vi "MintDAQ_Beta.vi"() -> ()   [LabVIEW 2016]
panel:
  in  "Cap 1":bool
  in  "Cap 2":bool
  in  "Freq":dbl=0.01
  in  "Amplitude 2":dbl
  in  "Amplitude":dbl=0.8
  in  "Freq":dbl=23.0
  in  "Write Rate":dbl=10.0 caption="dt"
  in  "Sampling Rate":dbl=40000.0
  in  "Buffer Size":i32=4000
  in  "Write":bool
  in  "?":T1(tab)=enum."Tiltmeters"
  out "Autocollimator":dynamicdata(graph)=[{"t0"=timestamp(3584301002.5607347 s since 1904-01-01), "dt"=0.001, "Y"=[0.43344412524716275, 0.44069982519207607, 0.43655847876988113, 0.42350642292314034, 0.4146197136070306, 0.40328027718902293, 0.39942297611809274, 0.4138427514859054, 0.43133329303091206, 0.4401128151072484, 0.43836303037775065, 0.4268035667025681, 0.41776134669103937, 0.4081520871618321, 0.3973264314407923, 0.40451695532239695, 0.42365021840797523, 0.4371180164475837, 0.44051733088947315, 0.43218711118964986, 0.4199243425497037, 0.41144729607965697, 0.40023572923979245, 0.40256453255522423, 0.4201710092812293, 0.43540959521302963, 0.44061842403674967, 0.43514094770763817, 0.4229076947032227, 0.41542396512922825, 0.4036505189077752, 0.39764993036831303, 0.41128629312723475, 0.42947942407640227, 0.4393467955648082, 0.439042631598667, 0.4271195679597182, 0.4169354468917369, 0.40734018701660385, 0.39899684628439686, 0.4082397862434385, 0.4262945383060813, 0.43778423869402877, 0.43953504788495423, 0.43013073777755223, 0.4190052781090954, 0.4114736084618774, 0.39912033284721876, 0.39913511226819326, 0.41637529988773103, 0.4326674073674492, 0.43974541690406393, 0.43570297775219, 0.4228391823041936, 0.4140567272130008, 0.402701353056287, 0.3991090457834896, 0.4137770345418973, 0.43097323181603453, 0.4394470896782597, 0.4377942918071419, 0.4263116695710484, 0.4171272850724305, 0.4075348167671378, 0.3970839223594497, 0.4044637556449303, 0.4233829165327582, 0.43680544817756956, 0.4402300393978032, 0.4319166495398041, 0.41960570181479623, 0.4111593303392392, 0.40019476380839447, 0.40300233950678993, 0.42065135304062434, 0.4355014297003315, 0.44083554591542506, 0.4351436898724957, 0.4227202848683051, 0.41516835962986626, 0.4036343684260499, 0.39781155478525676, 0.4113785124281454, 0.42957368340023233, 0.4395899330139984, 0.43921976442080857, 0.4276083237349742, 0.4171979089612628, 0.40734771090408123, 0.39878896340014114, 0.40840145058911986, 0.4268058170469636, 0.4388983111642708, 0.4406845835982937, 0.43145885626559677, 0.4203370587721238, 0.41243669736511696, 0.39995864936217074, 0.40047445740636817, 0.41809542489158874], "attributes"=variant("NI_ChannelName"=variant(string "Voltage_0 (Resampled)"), "NI_OriginalChannelName"=variant(string "Voltage_0"), "NI_UnitDescription"=variant(string "Volts"))}, {"t0"=timestamp(3584301002.5607347 s since 1904-01-01), "dt"=0.001, "Y"=[-0.4899930623675261, -0.49618517779377413, -0.49147473661274943, -0.47916473468257553, -0.4704209717410225, -0.4582103112231087, -0.4526439182566501, -0.4659935832899469, -0.48455155517052584, -0.49424384784604775, -0.4932876028975129, -0.4820006431763008, -0.4713454192343676, -0.46126420772334953, -0.4526272342865088, -0.4612194371103458, -0.4797607607514805, -0.49302166652545454, -0.49521427664385614, -0.4868851477690577, -0.47533904868769833, -0.46672055134251855, -0.4541546185640615, -0.45500585120320913, -0.47242507473390616, -0.48873125108294935, -0.4945101576910096, -0.4899985184460449, -0.47743833204721203, -0.4681475657146796, -0.4568603632196832, -0.45348452666153055, -0.4676122352684016, -0.4854852393103641, -0.49448520869432916, -0.4929760361070191, -0.48215125593273594, -0.4724288980813809, -0.46230160185882047, -0.45255984568019675, -0.4603440066276953, -0.4790831606691835, -0.49193190119468344, -0.4939058046810938, -0.485233635661633, -0.47322045802489393, -0.4644010543949078, -0.45350452925151147, -0.4555514886382289, -0.47263933075512876, -0.4889300758093243, -0.4950357596717817, -0.49031038481930594, -0.47827199879209714, -0.46999509979188464, -0.4577384596085571, -0.45219785195499623, -0.4659456404234807, -0.4845318190554642, -0.4940755974102945, -0.49312101619460347, -0.4816196861704534, -0.471090372935818, -0.46103550206715527, -0.45263650825676627, -0.46137101942036873, -0.4798528078286872, -0.49313741198078714, -0.49543043621354604, -0.48695040146175766, -0.4754215207234197, -0.4669228011335708, -0.45462597451738224, -0.455656611737308, -0.4731293161972794, -0.4894979885994622, -0.4952040342980257, -0.4902406511721809, -0.4774719474264416, -0.46846835181803426, -0.45710476738836775, -0.4538789376280827, -0.4679295376321548, -0.4857340010820316, -0.4952446398898893, -0.4941617238524955, -0.48283552180991424, -0.472828386804153, -0.46237264355045776, -0.45247223540877285, -0.4605043030686478, -0.4795100791768031, -0.4928472486855602, -0.4951132365031468, -0.4866591336331644, -0.4744833451831475, -0.4653165753980979, -0.45402960545544296, -0.4567301182540441, -0.47430536603009305], "attributes"=variant("NI_ChannelName"=variant(string "Voltage_1 (Resampled)"), "NI_OriginalChannelName"=variant(string "Voltage_1"), "NI_UnitDescription"=variant(string "Volts"))}, {"t0"=timestamp(3584301002.5607347 s since 1904-01-01), "dt"=0.001, "Y"=[0.4752534068648039, 0.4828089160742462, 0.4788214769070343, 0.46572582080473335, 0.4565461791038042, 0.4443905362197303, 0.44000211116761917, 0.45503506545430505, 0.4729492304645799, 0.48202113067256525, 0.4808637091287431, 0.46920339337455635, 0.459935061678949, 0.44976240866428896, 0.4380479127034327, 0.4452268064842056, 0.46481582898769525, 0.47880170342650535, 0.48264420637467514, 0.4743906358277276, 0.46191057491608306, 0.4530840898894057, 0.4412318111486498, 0.4435215400985711, 0.46159457744762983, 0.477019787853237, 0.48255506818894933, 0.4772042494056515, 0.4648366957946227, 0.4573035093760146, 0.4449690262346409, 0.4381851188092257, 0.4520426997895871, 0.4709815651668292, 0.48115794076123564, 0.48112845083648254, 0.4694327073406184, 0.45888006844449786, 0.4487109118407287, 0.4395954454135707, 0.4492612853971449, 0.46794570620513515, 0.4798195763650816, 0.48151531103537404, 0.4724718956854497, 0.46126640623768145, 0.4533215340906096, 0.4400094793568389, 0.43962361572182707, 0.45724133993585503, 0.47407933524264184, 0.4817390509485612, 0.47814826426104107, 0.46512671712574083, 0.4558880569960872, 0.4438023941344438, 0.43981420179845593, 0.45493875604870854, 0.47251009857461485, 0.48149700806397755, 0.4801525843124307, 0.46851761572489187, 0.4592185111821079, 0.449107151166732, 0.4377481013634747, 0.445126787340761, 0.4647276210890167, 0.4786996491590686, 0.4825017668160714, 0.47414042594077266, 0.4617773738849871, 0.4528292667611211, 0.44104227652050243, 0.44397723860813226, 0.46206847167797016, 0.47744680199800166, 0.482904801169116, 0.4773367538146408, 0.4648981271291952, 0.4572110463365532, 0.4447038387899914, 0.4381429239312602, 0.4521789849056913, 0.47116042336556857, 0.48153309131277666, 0.4816012687760707, 0.46984090928218913, 0.45923197895345846, 0.4488122671488527, 0.4395189501881836, 0.4492260144608356, 0.4683041316217303, 0.4807697375573159, 0.48295048700141024, 0.4739386073659291, 0.4626122471257542, 0.45423849004920125, 0.44080911543567924, 0.4410275575529489, 0.4590714921116883], "attributes"=variant("NI_ChannelName"=variant(string "Voltage_2 (Resampled)"), "NI_OriginalChannelName"=variant(string "Voltage_2"), "NI_UnitDescription"=variant(string "Volts"))}, {"t0"=timestamp(3584301002.5607347 s since 1904-01-01), "dt"=0.001, "Y"=[-0.46741716497017777, -0.47335196640769966, -0.4688101106381729, -0.45664050832791825, -0.448213130229613, -0.43623637113558433, -0.4302350320045326, -0.443538767561202, -0.4620528306577105, -0.47180156044258226, -0.4708179292756164, -0.45932138214803, -0.44882444701322133, -0.4389473643137334, -0.43021263768566703, -0.4389290270042119, -0.45719365582869087, -0.4703195255934425, -0.4725062586174858, -0.46412351904437593, -0.45266599902163945, -0.44452929290396437, -0.43224727493757303, -0.433114799318174, -0.45019875498394113, -0.46635052962592644, -0.4719961600068473, -0.46714017408877456, -0.4545566334501105, -0.4457455334827045, -0.4346493726108762, -0.43132205254719647, -0.44530002650432604, -0.46285119812847075, -0.47207996069808766, -0.47059195488018213, -0.45955848571273333, -0.4500080560551608, -0.4401595273597742, -0.4301296000567366, -0.43801005748286365, -0.4566340086643006, -0.46948052785402705, -0.4715299136445929, -0.46296642056819104, -0.4510050717407777, -0.4421868675692818, -0.4312254572681137, -0.43334469002882126, -0.4502249766779762, -0.4663893185758022, -0.4723950091453868, -0.4677093870036369, -0.4556402366748204, -0.44762001610851043, -0.43565467909521993, -0.43006135245785876, -0.4436904043107216, -0.4620902280747182, -0.47142412511475446, -0.47024445029591094, -0.4589520553752298, -0.4485546596952788, -0.43859895643507807, -0.4306030776532733, -0.4393468653762087, -0.45741650230252456, -0.4704208110651226, -0.47263895113144194, -0.46421030635564, -0.4527845970734405, -0.444608571264416, -0.432363860493319, -0.4334958061593289, -0.45081792059554604, -0.46707088362812127, -0.4726735792855328, -0.46757879668582364, -0.4548368413126195, -0.4460545704137894, -0.43474301847712926, -0.43137276244766654, -0.445408995733169, -0.46311295892705107, -0.4725715287342226, -0.47153021415590585, -0.4602416931812259, -0.45035976038962683, -0.44019822805303566, -0.4301401207313045, -0.438126286596999, -0.4570490190948041, -0.4702425601487558, -0.472657799778612, -0.4639172885988271, -0.45188581974347247, -0.44311506846835363, -0.43191775344563943, -0.43456605480841076, -0.45198857446235324], "attributes"=variant("NI_ChannelName"=variant(string "Voltage_3 (Resampled)"), "NI_OriginalChannelName"=variant(string "Voltage_3"), "NI_UnitDescription"=variant(string "Volts"))}]
  out "Interferometer":dynamicdata(graph)=[{"t0"=timestamp(3584301002.6527343 s since 1904-01-01), "dt"=0.001, "Y"=[0.006829190660454283, 0.006804074276043003, 0.006842802827010677, 0.0068415847383131246, 0.006839182378433872, 0.00685776770236201, 0.0068254281770467815, 0.00679490793515514, 0.006826136166008299, 0.006839250927218066, 0.006885744974215802, 0.006872920153230099, 0.0068459556593170635, 0.0067788572277271844, 0.006810908798271245, 0.006843586682920005, 0.006844003743632374, 0.006861160983203973, 0.006829789230096557, 0.006814916139960706, 0.006791236131882309, 0.006763083615057042, 0.006819530591850722, 0.006824557604947039, 0.006798398078015609, 0.006804774029728807, 0.0068032101016440956, 0.006765665610306133, 0.006752128475637698, 0.006839443300822217, 0.006760255089729292, 0.006741599354218663, 0.00678611945914091, 0.006790148597221571, 0.006765265780400054, 0.006733891478046875, 0.006749705918959564, 0.006678182149209056, 0.006674296646808111, 0.006718840100145775, 0.006716051786096207, 0.006700679563828491, 0.006744182507010799, 0.006789261097002876, 0.006718023450393194, 0.006733849047081241, 0.006768159078276218, 0.00670562987110903, 0.0067931254919439184, 0.006766590257329877, 0.006757634195636475, 0.006738605612389788, 0.006738138892240513, 0.0067589991043940836, 0.006799606400498515, 0.006810258091940859, 0.006745698101846311, 0.0067758918641107795, 0.0067580007161438735, 0.006784504446825061, 0.0067947629744846885, 0.006759420468503427, 0.006807751744288853, 0.006844330204419778, 0.006796933133234253, 0.006767604642546505, 0.006800642686309006, 0.00680934660333741, 0.006797574852825216, 0.006818358205769789, 0.006796135078595576, 0.006797976710975998, 0.00682167125723123, 0.0068453855491922636, 0.00683078505894028, 0.006816237213630237, 0.006836766164359942, 0.006830055877761378, 0.006809951504255314, 0.006879278069927046, 0.006828506557633108, 0.006796904922860819, 0.00678984148192317, 0.0068003542314009615, 0.006781409933802676, 0.006768389062226075, 0.0068260796398966535, 0.006782028912536799, 0.006763515121172703, 0.006736620043527606, 0.0067113376652639615, 0.006758038372946205, 0.006762727514682312, 0.006764384225255027, 0.006715498251011387, 0.006724243652234973, 0.0066958975856384, 0.006695695525440389, 0.0067368957309638785, 0.006717783312505214], "attributes"=variant("NI_ChannelName"=variant(string "Voltage_0 (Resampled)"), "NI_OriginalChannelName"=variant(string "Voltage_0"), "NI_UnitDescription"=variant(string "Volts"))}, {"t0"=timestamp(3584301002.6527343 s since 1904-01-01), "dt"=0.001, "Y"=[0.014079520299369902, 0.014089443536113735, 0.01413838279236252, 0.014073268951156152, 0.01406504585971624, 0.014094152205166504, 0.014076717713778275, 0.01410976032104998, 0.014083340578053195, 0.014083047059254608, 0.014073947149022274, 0.014145253440018832, 0.014094260993791834, 0.0140712503491944, 0.014059874273873623, 0.01405289434036577, 0.014047340666948032, 0.01409862304928333, 0.0140780703598332, 0.014092916485748829, 0.01404770682724726, 0.014088107561823415, 0.014062112790610122, 0.014041402834955993, 0.014071921491964982, 0.014043025726374177, 0.014073195489615439, 0.014063407668480674, 0.014092498018178494, 0.014058393522085606, 0.01405821946350781, 0.014034068491767523, 0.014046707469062806, 0.014052762554210126, 0.014121276368777845, 0.01407928275169214, 0.014016736267355124, 0.014002637471172086, 0.014004770641207642, 0.014010865997918256, 0.014038106702091477, 0.014000388730206906, 0.014003110570523036, 0.014035772574007713, 0.014015678283132122, 0.013995996432146158, 0.014014366493847085, 0.01402938421206668, 0.014017085207530632, 0.014054635185166007, 0.014038340870197532, 0.014069513721362708, 0.014031123864759243, 0.01402892779888155, 0.014061224413235873, 0.01404060636115332, 0.014044978845244149, 0.013997494228631023, 0.014071469993759932, 0.014062308683913503, 0.014075231637268865, 0.014074931537452704, 0.014091680839285385, 0.014096028326234987, 0.01412212044842212, 0.014084767395675726, 0.014031174341889817, 0.014017825746510044, 0.014019425281673164, 0.014027138319086589, 0.01401270152711483, 0.014097329823873036, 0.014108779023646675, 0.014042530650638322, 0.014032682296044144, 0.014098057535918914, 0.014032398902387104, 0.014054667811692102, 0.014052980427935688, 0.01412931155397704, 0.014098718955442072, 0.014095034956812436, 0.014049628590867239, 0.014093437040998746, 0.014071326434821394, 0.014055944856256063, 0.01402078171243926, 0.014052632057341656, 0.014048405726922885, 0.014081409428061308, 0.014003006477915724, 0.014049046467740472, 0.014007229224388525, 0.014063501022372934, 0.014139246375744385, 0.014061430667785901, 0.014079495475464476, 0.014006584025108057, 0.014038461617348556, 0.014020381795830343], "attributes"=variant("NI_ChannelName"=variant(string "Voltage_1 (Resampled)"), "NI_OriginalChannelName"=variant(string "Voltage_1"), "NI_UnitDescription"=variant(string "Volts"))}]
  out "Y-Tilt":dynamicdata(graph)
  out "X-Tilt":dynamicdata(graph)
  out "Interferometer Angle":dynamicdata(graph)=[{"t0"=timestamp(3584301002.652747 s since 1904-01-01), "dt"=0.001, "Y"=[0.014079523842758108, 0.01408882108377099, 0.014139037672450625, 0.01407280813247636, 0.014064729768797652, 0.014093702444871162, 0.014076359649149703, 0.01411085646219041, 0.014083787524917802, 0.014082287987847044, 0.014074911580000458, 0.014144148120125894, 0.01409290939216138, 0.014071860270478593, 0.014057498877325273, 0.014053501645067348, 0.014047463627659731, 0.014099356512726424, 0.0140787455400635, 0.01409152835182853, 0.014049362307693625, 0.014087897830537143, 0.0140614757950326, 0.014042240804392111, 0.014070969369652558, 0.014044862257688149, 0.014073507734953052, 0.014063096601953953, 0.014092704610592833, 0.014057846494315143, 0.014057636810089123, 0.014033601584274325, 0.014047269712564809, 0.014054091284079504, 0.014121881593934958, 0.014078136875977384, 0.014017481543910942, 0.014002358090528645, 0.01400554546932183, 0.014010414955054694, 0.014038264896493648, 0.013999825279258285, 0.01400260275898491, 0.01403404230826596, 0.014015566872301042, 0.01399606172889438, 0.01401524513663883, 0.01402868894874523, 0.014017869341953869, 0.014053872816437472, 0.014039558372932455, 0.014068713483619042, 0.014032643875552408, 0.01402809579860335, 0.014061676497261831, 0.014041263242768722, 0.014044765126358884, 0.013998027952526065, 0.014072116056769167, 0.014062055203707482, 0.014076231461729122, 0.014075052887551096, 0.014091733649736803, 0.014096658086670839, 0.014121966803459183, 0.014085631910137323, 0.014030455531931753, 0.014017122443594274, 0.01401924157308815, 0.014027275362907635, 0.014013742246393297, 0.014098782021426151, 0.014108111501473146, 0.01404194075891019, 0.014033749910072535, 0.01409771047400392, 0.014031347764116115, 0.014054660423562678, 0.014053518858002158, 0.014129918899766608, 0.01409814111093245, 0.014094692849691937, 0.014049505711538837, 0.014094509569479151, 0.014072003851555298, 0.01405603645142166, 0.014020787548272127, 0.014051507739459205, 0.01404965592418739, 0.014080831673375952, 0.01400344836335159, 0.014048947686481078, 0.014007080419140387, 0.014064113346367164, 0.014138793541416384, 0.014060465784733089, 0.014079431005924018, 0.01400604029938445, 0.014038771619406138, 0.01402036849841128], "attributes"=variant("NI_ChannelName"=variant(string "Voltage_1 (Resampled)"), "NI_OriginalChannelName"=variant(string "Voltage_1"), "NI_UnitDescription"=variant(string "Volts"))}]
  out "Autocollimator Angle":dynamicdata(graph)=[{"t0"=timestamp(3584301002.5607347 s since 1904-01-01), "dt"=0.001, "Y"=[-0.05451833877723473, -0.05477533979676578, -0.05480582827131981, -0.054733234251106065, -0.05438452166115732, -0.05328249062231282, -0.05282928135642799, -0.05380742715640242, -0.05429267469512887, -0.05453029541879096, -0.055158108535643346, -0.05495324117150584, -0.054737105032500843, -0.05390617367682065, -0.05287580869831008, -0.053150091215801595, -0.05375844613293926, -0.054305489087989864, -0.05474256186511284, -0.05468787010309875, -0.054464146880406406, -0.053980763474418665, -0.05319596601622297, -0.05341507708546636, -0.05409286356894648, -0.05423308435586057, -0.05452651489614367, -0.05453725909672287, -0.05437428211257543, -0.05433893468520682, -0.053531422557000344, -0.052740294552652806, -0.053250414130049384, -0.05415371986656394, -0.05442042116671404, -0.05463111639248197, -0.05482945152523553, -0.05442711090661558, -0.053612604169809015, -0.05276062517907868, -0.05356674134825469, -0.054364647974460806, -0.05473078730661945, -0.054529266336172895, -0.054872106202178986, -0.05484029684965096, -0.05424943872507388, -0.053020503666677266, -0.05278046062927735, -0.05338179240033376, -0.05399934610464124, -0.05462878331890356, -0.0550440444000253, -0.05482138827862627, -0.0542636140340086, -0.053271217757039795, -0.05299800290380298, -0.0537637882823139, -0.054184528206733, -0.05471748678812945, -0.05496820360224187, -0.05470350277314279, -0.05463311899197042, -0.05386273864045209, -0.052807622422947814, -0.053089720433317195, -0.0539894738939846, -0.05458084492323193, -0.05492879411526293, -0.05471494807201495, -0.05470264547182372, -0.05401921708034396, -0.053004545381501254, -0.05344398804351714, -0.05408676006037784, -0.054669368635636456, -0.05469729224640852, -0.05470551107247462, -0.05470159312764469, -0.054550536191225144, -0.053211554910672726, -0.05248128758956602, -0.05330129496244606, -0.054265667488309556, -0.054598057744387876, -0.05501212395163068, -0.054721672453989546, -0.05453950323691921, -0.053729192585936156, -0.05293366875685083, -0.05331091185378958, -0.05417210090301452, -0.05452392463979469, -0.05490399470516479, -0.05505330134879471, -0.05485221959895576, -0.05418344956409292, -0.05297257260307909, -0.052866907118601585, -0.053531331100620604], "attributes"=variant("NI_ChannelName"=variant(string "Voltage_0 (Resampled)"), "NI_OriginalChannelName"=variant(string "Voltage_0"), "NI_UnitDescription"=variant(string "Volts"))}, {"t0"=timestamp(3584301002.5607347 s since 1904-01-01), "dt"=0.001, "Y"=[0.029184874400107766, 0.029669964725631895, 0.02960380431772896, 0.029435387639123962, 0.028980595921586996, 0.028729684540872866, 0.02907643674907737, 0.028940253349997197, 0.029047499543346057, 0.029121962095730525, 0.02928959942345358, 0.029655428059348773, 0.02938076977263026, 0.029178858486904546, 0.02915843360419281, 0.02875499375154043, 0.029106053892906436, 0.029415157932796126, 0.029558825682914916, 0.029748360244639466, 0.02959070887957728, 0.02900148552377682, 0.02859649573632491, 0.028310538126707523, 0.028644755566355724, 0.028940618187186348, 0.029250973456318403, 0.02985522336081171, 0.02990198150552743, 0.029240394970527935, 0.02901526563556768, 0.02873266721257002, 0.028754890186645187, 0.0292319062945649, 0.029087666241611947, 0.029182614070472436, 0.029528950578401207, 0.029237856496264477, 0.028956988429858374, 0.02920088778390613, 0.02882022760087491, 0.028949607052927588, 0.029094541405657818, 0.02912515043959512, 0.029120149635372572, 0.02900584976595074, 0.029022158842350463, 0.029053830542728892, 0.028718292497503038, 0.028892094164828703, 0.029149335140592206, 0.029417217514454235, 0.029514935252490913, 0.029565372123483882, 0.02919480164175955, 0.02887630452485412, 0.028722341227765128, 0.028675323472041703, 0.02897489544084521, 0.029392663289044496, 0.029824842326365376, 0.029637602227388652, 0.029397921351316653, 0.029331664893484953, 0.028662183913639065, 0.028415707636525275, 0.02893622093302352, 0.029429922855068385, 0.029665115737803532, 0.02972935630931994, 0.029547017836511737, 0.029165487232220108, 0.029055439836962058, 0.028655078231310156, 0.0287494884170076, 0.029010425976667573, 0.02928174068810139, 0.02959849853901873, 0.029571964958395675, 0.02925007905005125, 0.02921046706117887, 0.029185359628159907, 0.029032417421852738, 0.02921238635610886, 0.029425074046687212, 0.02950823327882449, 0.029541908662657133, 0.02930095588686082, 0.02900602253337073, 0.029065631981068485, 0.028872004576206735, 0.028962479142700916, 0.02928555170258849, 0.029224339721921764, 0.029737732695260113, 0.029505716148848084, 0.02901709012437195, 0.02883814858127603, 0.028648014906134667, 0.028758078332581812], "attributes"=variant("NI_ChannelName"=variant(string "Voltage_3 (Resampled)"), "NI_OriginalChannelName"=variant(string "Voltage_3"), "NI_UnitDescription"=variant(string "Volts"))}]
  in  "PID Input":bool
  out "Feedback":dynamicdata(graph)=[{"t0"=timestamp(3584301002.560747 s since 1904-01-01), "dt"=0.001, "Y"=[0.0, 0.0, 0.0, 0.0, 0.0, 0.0, 0.0, 0.0, 0.0, 0.0, 0.0, 0.0, 0.0, 0.0, 0.0, 0.0, 0.0, 0.0, 0.0, 0.0, 0.0, 0.0, 0.0, 0.0, 0.0, 0.0, 0.0, 0.0, 0.0, 0.0, 0.0, 0.0, 0.0, 0.0, 0.0, 0.0, 0.0, 0.0, 0.0, 0.0, 0.0, 0.0, 0.0, 0.0, 0.0, 0.0, 0.0, 0.0, 0.0, 0.0, 0.0, 0.0, 0.0, 0.0, 0.0, 0.0, 0.0, 0.0, 0.0, 0.0, 0.0, 0.0, 0.0, 0.0, 0.0, 0.0, 0.0, 0.0, 0.0, 0.0, 0.0, 0.0, 0.0, 0.0, 0.0, 0.0, 0.0, 0.0, 0.0, 0.0, 0.0, 0.0, 0.0, 0.0, 0.0, 0.0, 0.0, 0.0, 0.0, 0.0, 0.0, 0.0, 0.0, 0.0, 0.0, 0.0, 0.0, 0.0, 0.0, 0.0], "attributes"=variant("NI_ChannelName"=variant(string "Voltage_0 (Resampled)"), "NI_OriginalChannelName"=variant(string "Voltage_0"), "NI_UnitDescription"=variant(string "Volts"))}, {"t0"=timestamp(3584301002.560747 s since 1904-01-01), "dt"=0.001, "Y"=[-0.003049692667419053, -0.0030011632054061078, -0.002996518018028922, -0.0029827779629064987, -0.002969936113352624, -0.0029686840885194002, -0.0030714550816880013, -0.0031182601097152316, -0.0030961181067506215, -0.0030702960683242127, -0.0031556696339665167, -0.003056010712971206, -0.0029590470292609763, -0.0030446429366765533, -0.002998755886991544, -0.00289757201639633, -0.0029364950409000007, -0.0029978703214920866, -0.0030534579761776716, -0.00306865013859312, -0.003013746188494248, -0.002941985739241768, -0.002975215182450896, -0.0030736031997608475, -0.0031436370132216385, -0.003119638151751415, -0.00313688360069503, -0.003200363446943197, -0.003120515838852851, -0.0030992073779693096, -0.0030333548858917413, -0.002935256533575503, -0.002944937708864363, -0.003008774658902448, -0.0030689687797508373, -0.0030487168992998507, -0.003080560232342409, -0.002976009922175736, -0.002990476808699664, -0.002997972161262606, -0.0031482346201067296, -0.003215133385025752, -0.0031569483922634775, -0.003123058031455838, -0.0030834162651266045, -0.0031345660821078913, -0.0031593501896138776, -0.0030466035459227356, -0.0029823811664562356, -0.002966955667432815, -0.0030550137544457373, -0.0030121888939130233, -0.0030919653304827713, -0.0030764282655193578, -0.0030286548502291193, -0.002962715438738431, -0.0030469850748333807, -0.003143821683320151, -0.0031858434346675522, -0.0032726993185585433, -0.0031859175661686366, -0.0030983549242839655, -0.003126499096708473, -0.003154439027166124, -0.003051078595666944, -0.0029192029414693726, -0.0029795320910118933, -0.0030517968700238566, -0.0031078090437984766, -0.0030798043887342646, -0.002968772323109508, -0.00299256205978614, -0.0029752696012527694, -0.003065746078914158, -0.003142664871777985, -0.0031278285009034177, -0.003102616171912688, -0.003078624786513096, -0.003012176456560062, -0.0030685407894212925, -0.0030532677393301797, -0.0029440112864748194, -0.002839468055274482, -0.002955781919963107, -0.0030284792855605597, -0.002991621109287228, -0.0029662293652921628, -0.002934837279029464, -0.0029292499538955707, -0.0030142614762774973, -0.003142299723375851, -0.003094740857359699, -0.0030834498434977623, -0.003223813466166711, -0.0031622302883786233, -0.0031387689775952765, -0.0031624680902710553, -0.0030453733210472913, -0.002927372808287793, -0.00292036287756316], "attributes"=variant("NI_ChannelName"=variant(string "Voltage_4 (Resampled)"), "NI_OriginalChannelName"=variant(string "Voltage_4"), "NI_UnitDescription"=variant(string "Volts"))}, {"t0"=timestamp(3584301002.560747 s since 1904-01-01), "dt"=0.001, "Y"=[-0.0419451691736932, -0.04213397136367565, -0.042154391527895005, -0.04210039078733851, -0.04182406066280207, -0.040979425792335815, -0.04064575377650065, -0.04139845227224993, -0.04176552138001907, -0.041945875961085045, -0.04243495974688696, -0.04226950687152701, -0.04210445195558116, -0.04145475774024459, -0.04066738340557622, -0.04089095505973653, -0.041358847359998896, -0.041777527551470586, -0.042112761651914514, -0.04206654782148995, -0.041894063161484134, -0.04151425860188682, -0.04091468488219391, -0.041094128540214436, -0.0416144467008395, -0.04172172418310117, -0.041947643195890415, -0.04194504450699992, -0.04182399360111914, -0.04179189205963497, -0.041163298556466596, -0.04057226839332534, -0.040978484135791055, -0.04165521719640903, -0.041858489248501815, -0.042031969991565735, -0.04218032531260918, -0.04186697616857548, -0.041234925560187874, -0.0405799882220148, -0.041213879051893006, -0.04182506713537269, -0.042103762388083624, -0.04194632157334728, -0.042210231513215186, -0.04218009548111838, -0.04171713802069411, -0.040776902708704585, -0.04060867978652026, -0.041068744876227914, -0.04154361184666005, -0.04202848435433248, -0.042339163200905285, -0.04216588353396274, -0.04172787504367163, -0.040970386899929136, -0.040773365430044256, -0.04136304511733595, -0.041680931600763915, -0.04209776762485897, -0.04228342224083276, -0.04208181131018098, -0.04202843973054086, -0.0414254571804388, -0.04061494371421473, -0.04084394783327905, -0.041536638588880716, -0.04199400353439718, -0.042252954133303974, -0.04207980125627409, -0.04207292445054595, -0.041536161358252374, -0.04076991367817173, -0.04111832681371705, -0.04161322424789044, -0.04205551755409712, -0.04207491976463538, -0.04208079558385167, -0.042083216024666845, -0.04195632537604731, -0.04091868940555001, -0.04037317065188369, -0.041012020891848855, -0.041748708262008515, -0.04199883176583878, -0.04231918945121469, -0.042091065524704735, -0.04195788335179344, -0.04132179219068758, -0.04071692878925155, -0.04101304361525849, -0.04167341611429567, -0.04194659385006853, -0.042237546018531275, -0.04234773554837193, -0.042185084170227025, -0.04166361582372886, -0.04073714289884529, -0.040668900705412944, -0.0411887905747883], "attributes"=variant("NI_ChannelName"=variant(string "Voltage_0 (Resampled)"), "NI_OriginalChannelName"=variant(string "Voltage_0"), "NI_UnitDescription"=variant(string "Volts"))}, {"t0"=timestamp(3584301002.552747 s since 1904-01-01), "dt"=0.001, "Y"=[4.698558856944605e-06, 4.7042384185892055e-06, 4.675162549090393e-06, 4.689973323617886e-06, 4.6985804343707245e-06, 4.676409797307714e-06, 4.674852774949815e-06, 4.688802233997341e-06, 4.6912806572878e-06, 4.690052524075735e-06, 4.681342348104294e-06, 4.678288592925336e-06, 4.681037573939893e-06, 4.677931232195188e-06, 4.667534564698385e-06, 4.680664590919649e-06, 4.6924544748470255e-06, 4.670149948052578e-06, 4.670062309599805e-06, 4.676237222652673e-06, 4.666492909656395e-06, 4.6804157105122615e-06, 4.6871886831658706e-06, 4.6787444183540155e-06, 4.672749559758632e-06, 4.683738872036577e-06, 4.6630077375608405e-06, 4.657977036848412e-06, 4.676340571461413e-06, 4.700874197495369e-06, 4.69200456093008e-06, 4.698196222124365e-06, 4.685753924719665e-06, 4.682616863715975e-06, 4.678037258424881e-06, 4.6856936824801385e-06, 4.7020659695103085e-06, 4.682897907354301e-06, 4.702471991743499e-06, 4.685270732225905e-06, 4.6917773107079e-06, 4.6916108775713556e-06, 4.693880730462773e-06, 4.690245176248893e-06, 4.672587950542629e-06, 4.697889535228499e-06, 4.683440396462663e-06, 4.682546730759722e-06, 4.6916164315831145e-06, 4.683864725528507e-06, 4.697409380132391e-06, 4.6925340752527e-06, 4.691584514214445e-06, 4.6836452723541905e-06, 4.695694088268158e-06, 4.709697290250545e-06, 4.722568503764702e-06, 4.7009524756229445e-06, 4.685173101074728e-06, 4.682051079532445e-06, 4.701712532936734e-06, 4.682410760440411e-06, 4.683050718689626e-06, 4.663164494552434e-06, 4.687304587659254e-06, 4.695406112983935e-06, 4.680414416178407e-06, 4.69271982243097e-06, 4.689941558326997e-06, 4.689449896781862e-06, 4.69285229094534e-06, 4.679673743466315e-06, 4.6476534139927996e-06, 4.689067834928844e-06, 4.681949206553395e-06, 4.685045298025742e-06, 4.6860997041393756e-06, 4.666862811141036e-06, 4.655141263915157e-06, 4.667922440507146e-06, 4.663433957466344e-06, 4.677111243641375e-06, 4.6824597756597946e-06, 4.674640984086689e-06, 4.678432130249666e-06, 4.676092881061438e-06, 4.676925942360813e-06, 4.678860099784647e-06, 4.699454912900034e-06, 4.685755486753241e-06, 4.6874190169299055e-06, 4.680411876400209e-06, 4.69027949451859e-06, 4.68449302010556e-06, 4.677802336615631e-06, 4.707526014456434e-06, 4.689532594658673e-06, 4.691874093945714e-06, 4.678165342537276e-06, 4.70558607300561e-06], "attributes"=variant("NI_ChannelName"=variant(string "Voltage_1 (Resampled)"), "NI_OriginalChannelName"=variant(string "Voltage_1"), "NI_UnitDescription"=variant(string "Volts"))}]
  in  "Offset 1":dbl
  in  "Offset 2":dbl
  in  "AC Setpoint":dbl=-0.014
  in  "Gain":dbl
  in  "I term":dbl=0.01
  in  "Reset Button":bool
  in  "D term":dbl=60.0
  in  "Int Setpoint":dbl=0.00135
  # "Swing\nInjection"
  # "Torsion\nInjection"
  # "Interferometer"
  # "Autocollimator"
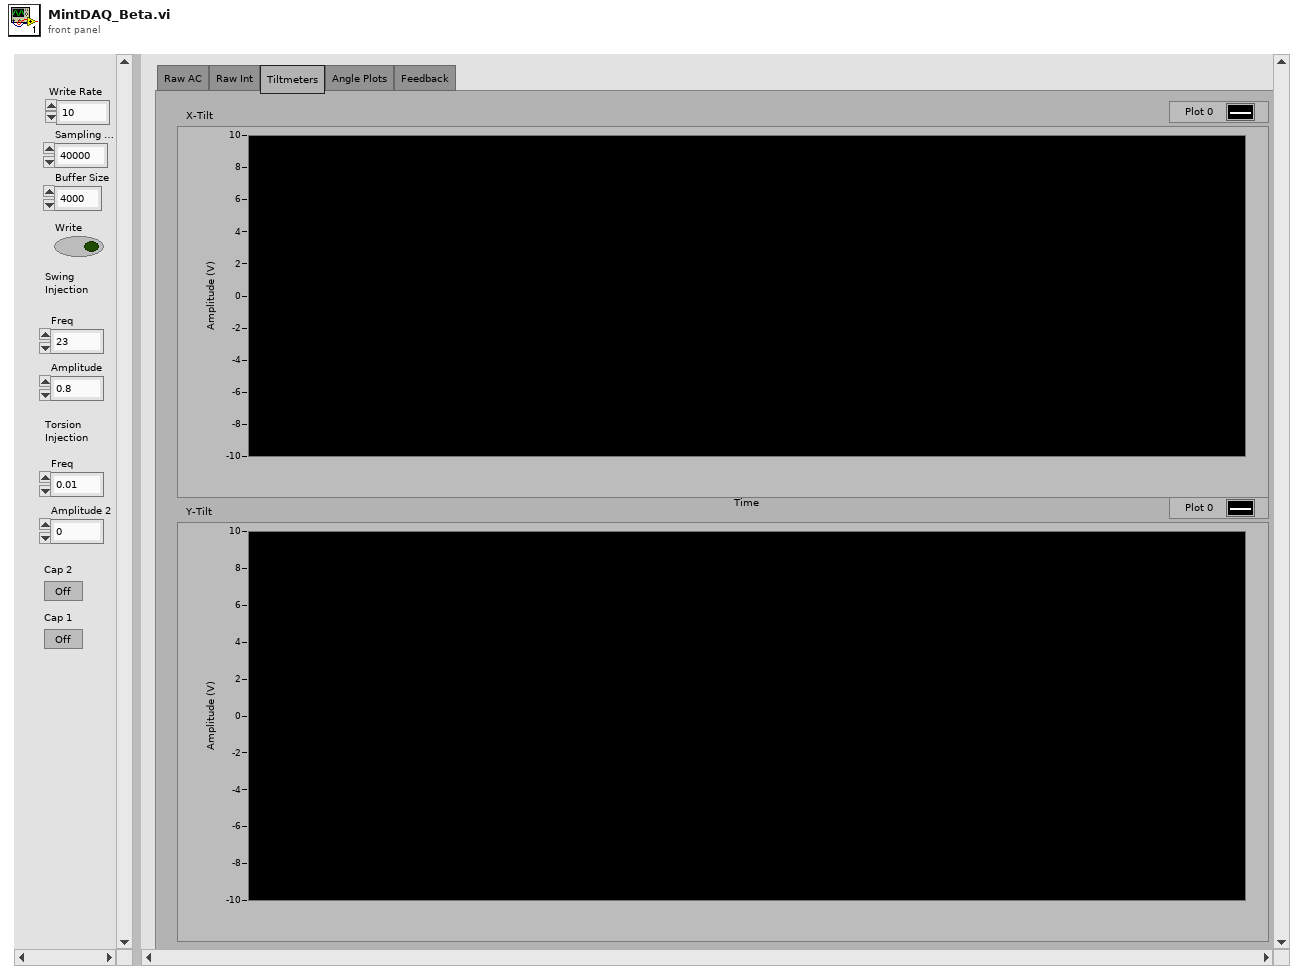
[diagram p1: front panel]
types:
  T1 = enum32{"Raw AC", "Raw Int", "Tiltmeters", "Angle Plots", "Feedback"}
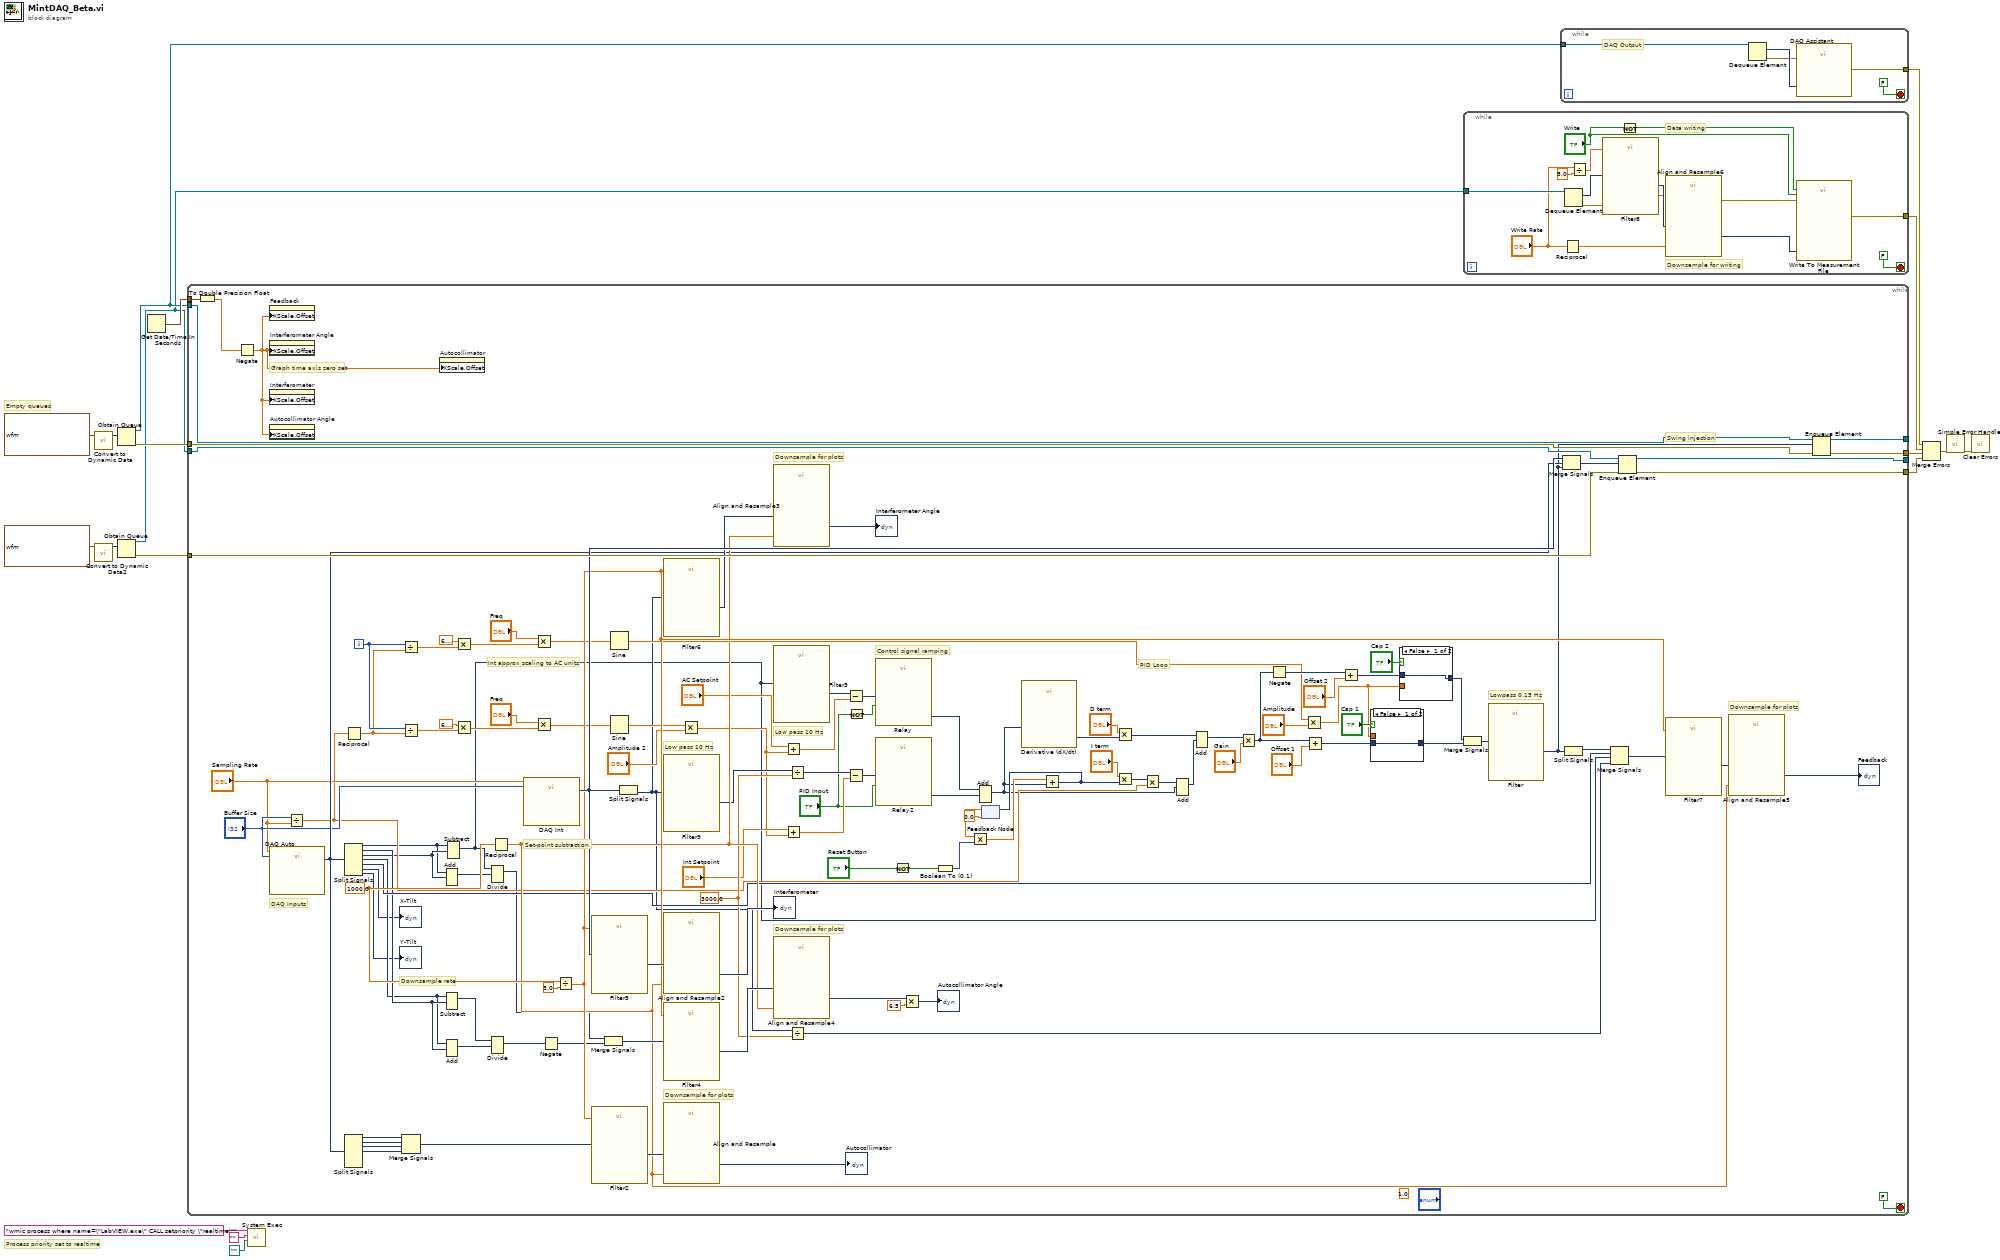
[diagram p0: block diagram]
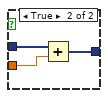
[diagram p2: hidden frame]
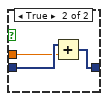
[diagram p3: hidden frame]
diagram:
  # "Empty queues"
  # "Process priority set to realtime"
  n1 = call "Convert to Dynamic Data"("Waveform"=waveform(dbl) {"t0"=timestamp(0 s since 1904-01-01), "dt"=1.0, "Y"=[]}) -> ("Dynamic Data Type"=w16:dynamicdata)  [unwired: 3 in]
  n2 = call "Convert to Dynamic Data2"("Waveform"=waveform(dbl) {"t0"=timestamp(0 s since 1904-01-01), "dt"=1.0, "Y"=[]}) -> ("Dynamic Data Type"=w14:dynamicdata)  [unwired: 3 in]
  n3 = Obtain Queue(element data type=w16) -> (queue out=w11:refnum<queue>, error out=w13:errorcluster)  [unwired: 4 in, 1 out]
  n4 = Obtain Queue(element data type=w14) -> (queue out=w10:refnum<queue>, error out=w12:errorcluster)  [unwired: 4 in, 1 out]
  n5 = Get Date/Time In Seconds() -> (seconds since 1Jan1904=w18:timestamp)
  n6 = while {
    tunnel: w18 -> [w136]
    tunnel: w11 -> [w133]
    tunnel: [w132] -> _
    tunnel: w10 -> [w116]
    tunnel: [w115] -> _
    tunnel: w13 -> [w114]
    tunnel: w12 -> [w113]
    tunnel: [w112] -> w8
    tunnel: [w111] -> w9
    i -> [w56]
    stop <- FALSE stop-if-true
    (unwired) 1.0 ("y")
    w92 = 3000.0 ("y")
    w96 = 1000.0 ("dt")
    # "Downsample for plots"
    # "Lowpass 0.15 Hz"
    # "PID Loop"
    # "Control signal ramping"
    # "Swing injection"
    # "Downsample rate"
    # "Downsample for plots"
    # "Downsample for plots"
    # "Downsample for plots"
    # "Int approx scaling to AC units"
    # "Set-point subtraction"
    # "Low pass 10 Hz"
    # "Low pass 10 Hz"
    # "DAQ Inputs"
    # "Graph time axis zero set"
    n7 = To Double Precision Float(number=w136) -> (double precision float=w135:dbl)
    n8 = Negate(x=w135) -> (-x=w134:dbl)
    n9 = property on="Feedback" class="WFChart (strict)"("XScale.Offset"=w134) -> ()  [unwired: 2 in, 2 out]
    n10 = property on="Interferometer Angle" class="WFChart (strict)"("XScale.Offset"=w134) -> ()  [unwired: 2 in, 2 out]
    n11 = property on="Interferometer" class="WFChart (strict)"("XScale.Offset"=w134) -> ()  [unwired: 2 in, 2 out]
    n12 = property on="Autocollimator Angle" class="WFChart (strict)"("XScale.Offset"=w134) -> ()  [unwired: 2 in, 2 out]
    n13 = call "DAQ Auto"("rate"="Sampling Rate", "number of samples"="Buffer Size") -> ("data"=w78:dynamicdata)  [unwired: 14 in, 3 out]
    n14 = Divide(x="Buffer Size", y="Sampling Rate") -> (x/y=w61:dbl)
    n15 = Split Signals(w78) -> (w83:dynamicdata, w82:dynamicdata, w81:dynamicdata, w80:dynamicdata)  [unwired: 7 in, 3 out]
    n16 = Split Signals(w78) -> (w26:dynamicdata, w31:dynamicdata, w27:dynamicdata, w30:dynamicdata, w94:dynamicdata, →"X-Tilt":dynamicdata, →"Y-Tilt":dynamicdata)  [unwired: 7 in]
    n17 = Reciprocal(x=w61) -> (1/x=w55:dbl)
    n18 = Divide(x=w56, y=w55) -> (x/y=w71:dbl)
    n19 = Divide(x=w56, y=w55) -> (x/y=w57:dbl)
    n20 = Merge Signals(w83, w82, w81, w80) -> (w79:dynamicdata)
    n21 = property on="Autocollimator" class="WFChart (strict)"("XScale.Offset"=w134) -> ()  [unwired: 2 in, 2 out]
    n22 = Add(1:w27, 2:w26) -> (0:w25:dynamicdata)  [unwired: 1 in, 1 out]
    n23 = Subtract(1:w31, 2:w30) -> (0:w28:dynamicdata)  [unwired: 1 in, 1 out]
    n24 = Add(1:w31, 2:w30) -> (0:w29:dynamicdata)  [unwired: 1 in, 1 out]
    n25 = Subtract(1:w27, 2:w26) -> (0:w21:dynamicdata)  [unwired: 1 in, 1 out]
    n26 = Multiply(x=6.283185307179586, y=w71) -> (x*y=w70:dbl)
    n27 = Multiply(x=6.283185307179586, y=w57) -> (x*y=w58:dbl)
    n28 = Divide(1:w25, 2:w21) -> (0:w24:dynamicdata)  [unwired: 1 in, 1 out]
    n29 = Divide(1:w29, 2:w28) -> (0:w23:dynamicdata)  [unwired: 1 in, 1 out]
    n30 = Reciprocal(x=w96) -> (1/x=w95:dbl)
    n31 = call "DAQ Int"("rate"="Sampling Rate", "number of samples"="Buffer Size") -> ("data"=w102:dynamicdata)  [unwired: 14 in, 3 out]
    n32 = Multiply(x="Freq", y=w70) -> (x*y=w68:dbl)
    n33 = Multiply(x="Freq", y=w58) -> (x*y=w59:dbl)
    n34 = Negate(x=w23) -> (-x=w22:dynamicdata)
    n35 = Divide(x=w96, y=3.0) -> (x/y=w97:dbl)
    n36 = call "Filter5"("Lower Cut-Off"=w97, "Signal"=w102) -> ("Filtered Signal"=w101:dynamicdata)  [unwired: 8 in, 1 out]
    n37 = call "Filter2"("Lower Cut-Off"=w97, "Signal"=w79) -> ("Filtered Signal"=w105:dynamicdata)  [unwired: 8 in, 1 out]
    n38 = Merge Signals(w24, w22) -> (w104:dynamicdata)
    n39 = Sine(x=w68) -> (sin(x)=w67:dbl)
    n40 = Sine(x=w59) -> (sin(x)=w60:dbl)
    n41 = Split Signals(w102) -> (w51:dynamicdata)  [unwired: 2 in, 1 out]
    n42 = call "Filter6"("Lower Cut-Off"=w97, "Signal"=w51) -> ("Filtered Signal"=w100:dynamicdata)  [unwired: 8 in, 1 out]
    n43 = call "Filter9"("Signal"=w51) -> ("Filtered Signal"=w50:dynamicdata)  [unwired: 9 in, 1 out]
    n44 = call "Align and Resample2"("dt"=w95, "Signals"=w101) -> ("Resampled Signals"=→"Interferometer":dynamicdata)  [unwired: 7 in, 2 out]
    n45 = call "Filter4"("Lower Cut-Off"=w97, "Signal"=w104) -> ("Filtered Signal"=w103:dynamicdata)  [unwired: 8 in, 1 out]
    n46 = call "Align and Resample"("dt"=w95, "Signals"=w105) -> ("Resampled Signals"=→"Autocollimator":dynamicdata)  [unwired: 7 in, 2 out]
    n47 = Multiply(x=w60, y="Amplitude 2") -> (x*y=w44:dbl)
    n48 = call "Align and Resample3"("dt"=w95, "Signals"=w100) -> ("Resampled Signals"=→"Interferometer Angle":dynamicdata)  [unwired: 7 in, 2 out]
    n49 = call "Filter3"("Signal"=w21) -> ("Filtered Signal"=w46:dynamicdata)  [unwired: 9 in, 1 out]
    n50 = call "Align and Resample4"("dt"=w95, "Signals"=w103) -> ("Resampled Signals"=w90:dynamicdata)  [unwired: 7 in, 2 out]
    n51 = Add(x="AC Setpoint", y=w44) -> (x+y=w47:dbl)
    n52 = Add(x="Int Setpoint", y=w44) -> (x+y=w49:dbl)
    n53 = Divide(x=w50, y=w92) -> (x/y=w48:dynamicdata)
    n54 = Divide(x=w51, y=w92) -> (x/y=w93:dynamicdata)
    n55 = Subtract(x=w46, y=w47) -> (x-y=w41:dynamicdata)
    n56 = Subtract(x=w48, y=w49) -> (x-y=w40:dynamicdata)
    n57 = Not(x="PID Input") -> (.not. x?=w36:bool)
    n58 = call "Relay"("Enable"=w36, "Signals"=w41) -> ("Result"=w38:dynamicdata)  [unwired: 8 in, 1 out]
    n59 = call "Relay2"("Enable"="PID Input", "Signals"=w40) -> ("Result"=w39:dynamicdata)  [unwired: 8 in, 1 out]
    n60 = Not(x="Reset Button") -> (.not. x?=w127:bool)
    n61 = Multiply(x=w90, y=6.5) -> (x*y=→"Autocollimator Angle":dynamicdata)
    n62 = Boolean To (0,1)(Boolean=w127) -> (0, 1=w85:i16)
    n63 = Add(1:w39, 2:w38) -> (0:w37:dynamicdata)  [unwired: 1 in, 1 out]
    n64 = feedback #1(0.0) -> (w87:dbl)
    n65 = Multiply(x=w87, y=w85) -> (x*y=w86:dbl)
    n66 = call "Derivative (dX/dt)"("Signals"=w37) -> ("Result"=w126:dynamicdata)  [unwired: 5 in, 1 out]
    n67 = Add(x=w86, y=w37) -> (x+y=w84:dynamicdata)
    n68 = feedback-in #1(w84) -> ()
    n69 = Multiply(x="D term", y=w126) -> (x*y=w124:dynamicdata)
    n70 = Multiply(x="I term", y=w84) -> (x*y=w77:dynamicdata)
    n71 = Multiply(x=w77, y=w61) -> (x*y=w75:dynamicdata)
    n72 = Add(1:w37, 2:w75) -> (0:w123:dynamicdata)  [unwired: 1 in, 1 out]
    n73 = Add(1:w123, 2:w124) -> (0:w122:dynamicdata)  [unwired: 1 in, 1 out]
    n74 = Multiply(x=w122, y="Gain") -> (x*y=w118:dynamicdata)
    n75 = Negate(x=w118) -> (-x=w119:dynamicdata)
    n76 = Multiply(x=w67, y="Amplitude") -> (x*y=w32:dbl)
    n77 = Add(x=w118, y="Offset 1") -> (x+y=w65:dynamicdata)
    n78 = Add(x=w119, y="Offset 2") -> (x+y=w63:dynamicdata)
    n79 = case shown="False" "Cap 1" {
      tunnel: w65 -> [w142 w145]
      tunnel: [w142 w144] -> w64
      tunnel: w32 -> [_ w143]
      frame False {
      }
      frame True {
        n80 = Add(x=w145, y=w143) -> (x+y=w144:dynamicdata)
      }
    }
    n81 = case shown="False" "Cap 2" {
      tunnel: w63 -> [w138 w141]
      tunnel: [w138 w140] -> w62
      tunnel: w32 -> [_ w139]
      frame False {
      }
      frame True {
        n82 = Add(x=w141, y=w139) -> (x+y=w140:dynamicdata)
      }
    }
    n83 = Merge Signals(w62, w64) -> (w43:dynamicdata)
    n84 = call "Filter"("Signal"=w43) -> ("Filtered Signal"=w42:dynamicdata)  [unwired: 9 in, 1 out]
    n85 = Merge Signals(w102, w78, w42) -> (w117:dynamicdata)
    n86 = Split Signals(w42) -> (w131:dynamicdata)  [unwired: 2 in, 1 out]
    n87 = Merge Signals(w131, w94, w21, w93) -> (w99:dynamicdata)
    n88 = Enqueue Element(queue=w116, element=w117, error in (no error)=w113) -> (queue out=w115:refnum<queue>, error out=w111:errorcluster)  [unwired: 1 in, 1 out]
    n89 = call "Filter7"("Lower Cut-Off"=w97, "Signal"=w99) -> ("Filtered Signal"=w98:dynamicdata)  [unwired: 8 in, 1 out]
    n90 = call "Align and Resample5"("dt"=w95, "Signals"=w98) -> ("Resampled Signals"=→"Feedback":dynamicdata)  [unwired: 7 in, 2 out]
    n91 = Enqueue Element(queue=w133, element=w42, error in (no error)=w114) -> (queue out=w132:refnum<queue>, error out=w112:errorcluster)  [unwired: 1 in, 1 out]
  }
  n92 = call <vilib>:"System Exec.vi"("working directory"=path "", "standard input"="", "command line"="wmic process where name=\"LabVIEW.exe\" CALL setpriority \"realtime\"") -> ()  [unwired: 5 in, 4 out]
  n93 = while {
    tunnel: w10 -> [w159]
    tunnel: [w146] -> w5
    stop <- FALSE stop-if-true
    # "Downsample for writing"
    # "Data writing"
    n94 = Reciprocal(x="Write Rate") -> (1/x=w155:dbl)
    n95 = Dequeue Element(queue=w159) -> (element=w157:dynamicdata, error out=w149:errorcluster)  [unwired: 2 in, 2 out]
    n96 = Divide(x="Write Rate", y=5.0) -> (x/y=w154:dbl)
    n97 = call "Filter8"("error in (no error)"=w149, "Lower Cut-Off"=w154, "Signal"=w157) -> ("error out"=w148:errorcluster, "Filtered Signal"=w158:dynamicdata)  [unwired: 7 in]
    n98 = Not(x="Write") -> (.not. x?=w150:bool)
    n99 = call "Align and Resample6"("dt"=w155, "error in (no error)"=w148, "Signals"=w158) -> ("error out"=w147:errorcluster, "Resampled Signals"=w156:dynamicdata)  [unwired: 6 in, 1 out]
    n100 = call "Write To Measurement File"("Signals"=w156, "Reset"=w150, "Enable"="Write", "error in (no error)"=w147) -> ("error out"=w146:errorcluster)  [unwired: 13 in, 2 out]
  }
  n101 = while {
    tunnel: w11 -> [w164]
    tunnel: [w161] -> w4
    stop <- FALSE stop-if-true
    # "DAQ Output"
    n102 = Dequeue Element(queue=w164) -> (element=w163:dynamicdata, error out=w162:errorcluster)  [unwired: 2 in, 2 out]
    n103 = call "DAQ Assistant"("data"=w163, "error in"=w162) -> ("error out"=w161:errorcluster)  [unwired: 16 in, 1 out]
  }
  n104 = Merge Errors(w4, w5, w8, w9) -> (w6:errorcluster)
  n105 = call <vilib>:"Simple Error Handler.vi"("error in (no error)"=w6) -> ("error out"=w7:errorcluster)  [unwired: 4 in, 4 out]
  n106 = call <vilib>:"Clear Errors.vi"("error in (no error)"=w7) -> ()  [unwired: 5 in, 2 out]
